vi "Call UI Initialize Device.vi"(8 "Error In":errorcluster) -> (0 "Error Out":errorcluster)   [LabVIEW 2019, in "Controller.lvlib"]
uses:
  Controller.lvlib
  Queues/Queues.lvlib
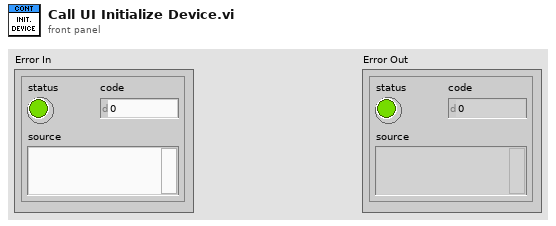
[diagram p1: front panel]
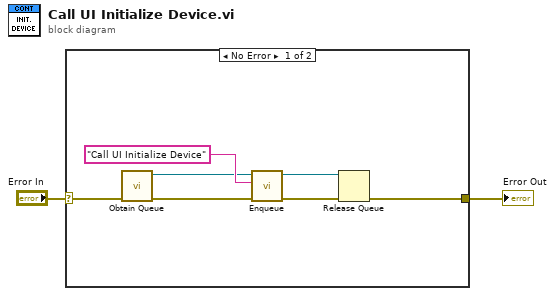
[diagram p0: block diagram]
diagram:
  n1 = case shown="No Error" "Error In" {
    selector: "Error In" -> [w8 w10]
    tunnel: [w3 w10] -> w2
    frame No Error {
      n2 = call "Obtain Queue.vi"("Error In"=w8) -> ("Error Out"=w7:errorcluster, "Queue out"=w6:refnum<queue>)  [unwired: 9 in]
      n3 = call "Enqueue.vi"("Error In"=w7, "State"="Call UI Initialize Device", "Queue in"=w6) -> ("Error Out"=w5:errorcluster, "Queue out"=w4:refnum<queue>)  [unwired: 7 in]
      n4 = Release Queue(queue=w4, error in (no error)=w5) -> (error out=w3:errorcluster)  [unwired: 1 in, 2 out]
    }
    frame Error {
    }
  }
  "Error Out" <- w2
